vi "imageNormalize.vi"(11 "Data":sgl[][](array[numeric])) -> (3 "Array":dbl[][](array[numeric]))   [LabVIEW 2021]
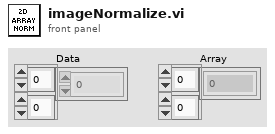
[diagram p1: front panel]
types:
  T1 = enum16{"nothing", "average", "8bit", "average/plane", "minimum", "plane", "average/stddev", "plane/average"}
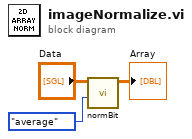
[diagram p0: block diagram]
diagram:
  n1 = call "normBit.vi"("method"=T1."average", "Rxy"="Data") -> ("Array"=→"Array":dbl[][])  [unwired: 8 in, 1 out]
